vi "Strain Configure Full Bridge Bend.vi"(4 "Channel":string, 5 "SampTime":dbl, 6 "SampCount":i32 format="%.0g", 7 "Range":dbl, 8 "error in (no error)":errorcluster {"code" format="%.0x"}, 9 "ExcitationVoltage":dbl, 10 "GaugeFactor":dbl, 11 "instrument handle":refnum<k15>) -> (0 "error out":errorcluster {"code" format="%.0x"}, 3 "instrument handle out":refnum<k15>)   [LabVIEW 2020, in "Keysight DAQ970.lvlib"]
doc: "Configures a specified channel for full bending bridge strain gauge DMM digitizing, but they do not initiate the digitizing. This command redefines the scan list."
uses:
  Keysight DAQ970.lvlib
  KtDAQ970.dll
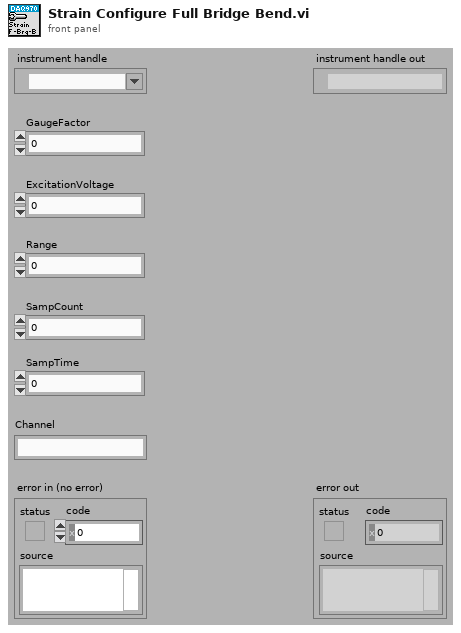
[diagram p1: front panel]
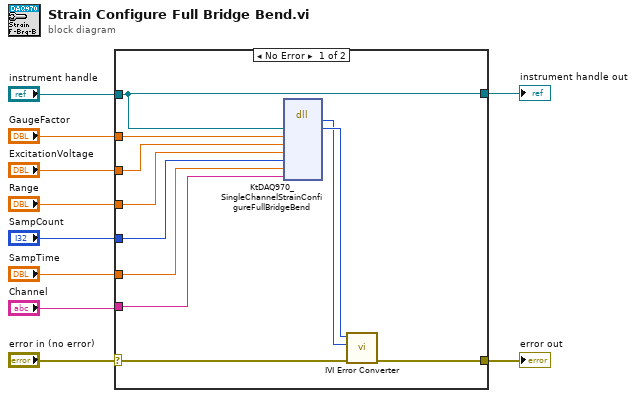
[diagram p0: block diagram]
diagram:
  n1 = case shown="No Error" "error in (no error)" {
    selector: "error in (no error)" -> [w19 w23]
    tunnel: [w18 w23] -> w10
    tunnel: "instrument handle" -> [w11 w22]
    tunnel: "GaugeFactor" -> [w17 _]
    tunnel: "ExcitationVoltage" -> [w16 _]
    tunnel: "Range" -> [w15 _]
    tunnel: "SampCount" -> [w14 _]
    tunnel: "SampTime" -> [w13 _]
    tunnel: "Channel" -> [w12 _]
    tunnel: [w11 w22] -> w1
    frame No Error {
      n2 = dll-call lib="KtDAQ970**.dll" fn="KtDAQ970_SingleChannelStrainConfigureFullBridgeBend"("Vi"=w11, "GaugeFactor"=w17, "ExcitationVoltage"=w16, "Range"=w15, "SampCount"=w14, "SampTime"=w13, "Channel"=w12) -> (w20:i32, "Vi"=w21:u32)  [unwired: 9 in, 2 out]
      n3 = call "IVI Error Converter.vi"("error in (no error)"=w19, "IVI error code (0)"=w20, "instrument handle"=w21) -> ("error out"=w18:errorcluster)  [unwired: 7 in, 1 out]
    }
    frame Error {
    }
  }
  "error out" <- w10
  "instrument handle out" <- w1
